vi "Car_Speed_R527.vi"(10 "精度":dbl=1.0, 11 "车速":u16) -> (3 "报文":T1 {"[7]" format="%02x"; "[6]" format="%02x"; "[5]" format="%02x"; "[4]" format="%02x"; "[3]" format="%02x"; "[2]" format="%02x"; "[1]" format="%02x"; "[0]" format="%02x"})   [LabVIEW 2020]
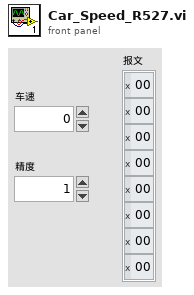
[diagram p1: front panel]
types:
  T1 = cluster{"[0]":u8, "[1]":u8, "[2]":u8, "[3]":u8, "[4]":u8, "[5]":u8, "[6]":u8, "[7]":u8}
  T2 = cluster{"y":u8, "y":u8, "y":u8, u8, u8, "y":u8, "y":u8, "y":u8}
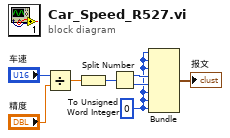
[diagram p0: block diagram]
diagram:
  w6 = u8 0 ("y")
  n1 = Divide(x="车速", y="精度") -> (x/y=w2:dbl)
  n2 = To Unsigned Word Integer(number=w2) -> (unsigned 16bit integer=w1:u16)
  n3 = Split Number(x=w1) -> (hi(x)=w8:u8, lo(x)=w7:u8)
  n4 = Bundle("y"=w6, "y"=w6, "y"=w6, w8, w7, "y"=w6, "y"=w6, "y"=w6) -> (→"报文":T2)  [unwired: 1 in]
